vi "Record Motor Values.vi"(8 "Target1 2":dbl format="%#_13g", 9 "Target1":dbl format="%#_13g", 10 "Motor Values":dbl[](array[numeric]), 11 "VI Block Name":string="Turn to Angle,") -> ()   [LabVIEW 2017]
uses:
  Robot Global Data.vi
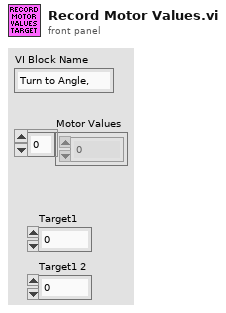
[diagram p1: front panel]
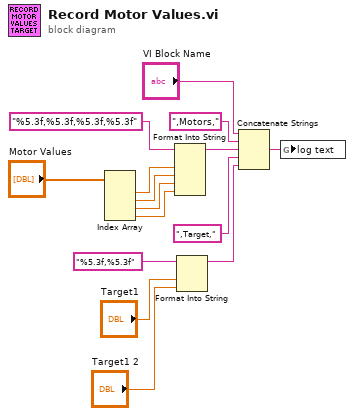
[diagram p0: block diagram]
diagram:
  n1 = Index Array(array="Motor Values") -> (element #1=w13:dbl, element #2=w11:dbl, element #3=w10:dbl, element #4=w9:dbl)  [unwired: 4 in]
  n2 = Format Into String(initial string="%5.3f,%5.3f,%5.3f,%5.3f", w13, w11, w10, w9) -> (resulting string=w7:string)  [unwired: 2 in, 1 out]
  n3 = Format Into String(initial string="%5.3f,%5.3f", "Target1", "Target1 2") -> (resulting string=w3:string)  [unwired: 2 in, 1 out]
  n4 = Concatenate Strings("VI Block Name", ",Motors," ("string"), w7, ",Target," ("string"), w3) -> (w15:string)
  n5 = global write "Robot Global Data.vi" "log text"(w15) -> ()
